vi "read-data-wfm-dvr.vi"(8 "error in (no error)":errorcluster, 11 "wfm dvr":refnum<data-value>) -> (0 "error out":errorcluster, 2 "Waveform":waveform(dbl))   [LabVIEW 2024]
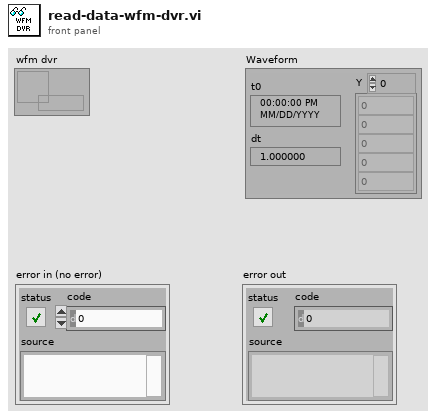
[diagram p1: front panel]
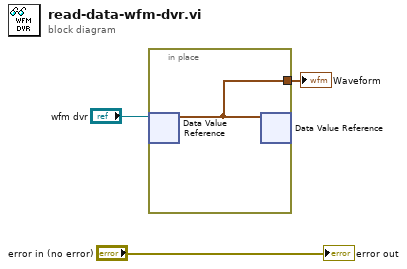
[diagram p0: block diagram]
diagram:
  n1 = in-place {
    in-place-border: [w4] -> w1
    n2 = in-place-dvr #1("wfm dvr") -> (w4:waveform(dbl))  [unwired: 1 out]
    n3 = in-place-dvr #1(w4) -> ()  [unwired: 2 out]
  }
  "Waveform" <- w1
  "error out" <- "error in (no error)"
